vi "AVItoArray.vi"() -> ()   [LabVIEW 2013]
panel:
  out "VideoArray":u8[][][](array[numeric])
  out "FrameSize":i32[](array[numeric])
  out "VideoArray Size":i32[](array[numeric])
  in  "Input video File":path=path "D:/RotationExperiments_v3_GCaMP6f+tdTomato/mouse013/session-m013-20161122-1807/labview_data/Block-11222016-1807-001-LightsON/EyeTracker-11222016-1807-001.avi"
  out "Number of Frames":u32
  out "FrameCounter":i32
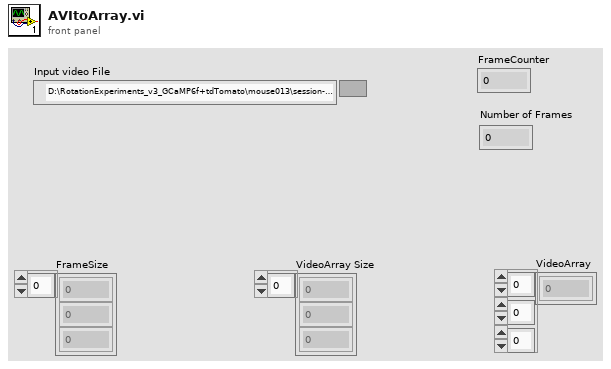
[diagram p1: front panel]
types:
  T1 = typedef "Image Type" = u32
  T2 = typedef "IMAQ AVI2 Refnum.ctl" = refnum<k20>
  T3 = typedef "IMAQ Image.ctl" = refnum<image>
  T4 = cluster{"Width":u32, "Height":u32, "Frames Per Second":u32, "Codec":string, "Has Data":bool}
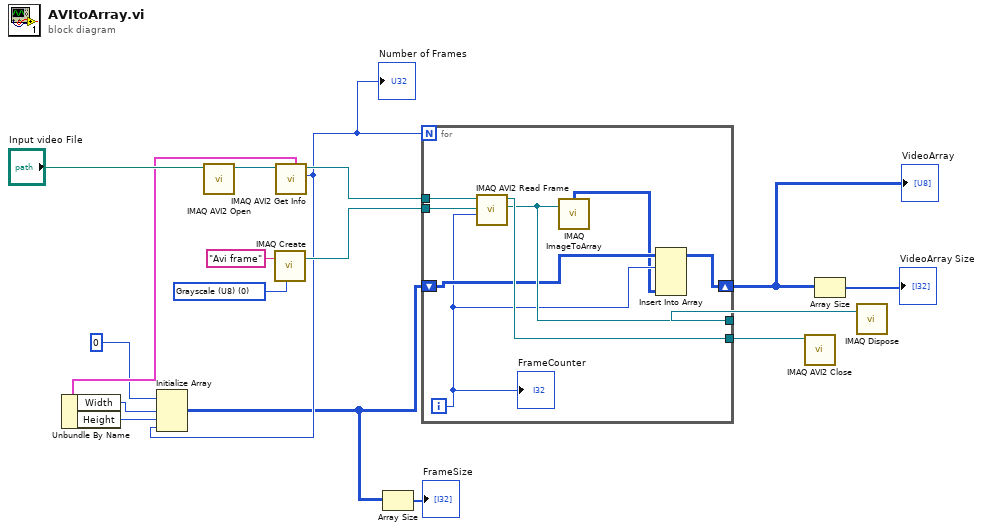
[diagram p0: block diagram]
diagram:
  w14 = T1 0 items=["Grayscale (U8)", "Grayscale (I16)", "Grayscale (SGL)", "Complex (CSG)", "RGB (U32)", "HSL (U32)", "RGB (U64)", "Grayscale (U16)"] ("Image Type")
  n1 = call "IMAQ AVI2 Open"("AVI File Path"="Input video File") -> ("AVI Refnum"=w16:T2)  [unwired: 9 in, 1 out]
  n2 = call "IMAQ Create"("Image Name"="Avi frame", "Image Type"=w14) -> ("New Image"=w12:T3)  [unwired: 3 in, 1 out]
  n3 = call "IMAQ AVI2 Get Info"("AVI Refnum"=w16) -> ("Number of Frames"=w4:u32, "AVI Refnum (duplicate)"=w13:T2, "Frame Data"=w7:T4)  [unwired: 6 in, 2 out]
  "Number of Frames" <- w4
  n4 = Unbundle By Name(w7) -> ("Width"=w6:u32, "Height"=w5:u32)
  n5 = Initialize Array(u8 0, w6, w5, w4) -> (w2:u8[][][])
  n6 = Array Size(array=w2) -> (size(s)=→"FrameSize":i32[])
  n7 = for {
    N: w4 -> [_]
    tunnel: w13 -> [w25]
    tunnel: w12 -> [w24]
    tunnel: [w23] -> w11
    tunnel: [w22] -> w10
    shift-right: [w20] -> w9
    shift-left: w2 -> [w21]
    i -> [w19]
    n8 = call "IMAQ AVI2 Read Frame"("Frame Number"=w19, "Image"=w24, "AVI Refnum"=w25) -> ("Image Out"=w22:T3, "AVI Refnum (duplicate)"=w23:T2)  [unwired: 6 in, 1 out]
    n9 = call "IMAQ ImageToArray"("Image"=w22) -> ("Image Pixels (U8)"=w18:u8[][])  [unwired: 3 in, 4 out]
    n10 = Insert Into Array(array=w21, index (dim 0)=w19, new element=w18) -> (w20:u8[][][])  [unwired: 2 in]
    "FrameCounter" <- w19
  }
  "VideoArray" <- w9
  n11 = call "IMAQ AVI2 Close"("AVI Refnum"=w11) -> ()  [unwired: 10 in, 1 out]
  n12 = Array Size(array=w9) -> (size(s)=→"VideoArray Size":i32[])
  n13 = call "IMAQ Dispose"("Image"=w10) -> ()  [unwired: 5 in, 1 out]
